vi "_add_attribute_name_to_error_message.vi"(7 "Attribute":T1={"Identifier"="", "Descriptive Name"="", "Data Type"=enum."Integer 32", "Command"="", "Access"=enum."Read/Write", "Range Table"="", "Read Callback"="", "Write Callback"="", "Supported Models"="", "Instrument Options"="", "Index"=0, "OPC Wait"=FALSE, "No Status Check"=FALSE, "Cache Only"=FALSE}, 8 "error in":errorcluster caption="error in (no error)", 10 "Recompose even if original message\nalready contains an attribute name (F)":bool, 11 "VISA resource name":refnum<visa-resource-name>) -> (0 "error out":errorcluster, 2 "Recomposed":bool, 3 "VISA resource name out":refnum<visa-resource-name>)   [LabVIEW 2022 SP3, in "hmp4000_rsidr_core.lvlib"]
uses:
  hmp4000_rsidr_core.lvlib
  type_Attribute.ctl
  type_Attribute_Data_Type.ctl
  type_ReadWriteAccess.ctl
  Trim Whitespace One-Sided.vi
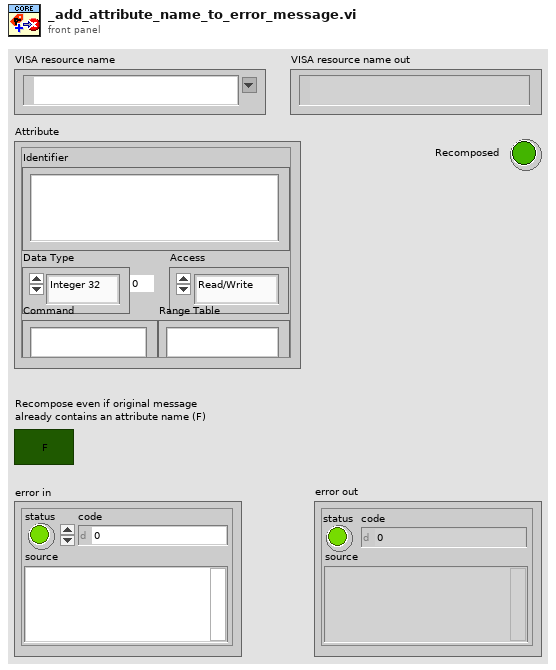
[diagram p1: front panel]
types:
  T1 = typedef "hmp4000_rsidr_core.lvlib/type_Attribute.ctl" = cluster{"Identifier":string, "Descriptive Name":string, "Data Type":T2, "Command":string, "Access":T3, "Range Table":string, "Read Callback":string, "Write Callback":string, "Supported Models":string, "Instrument Options":string, "Index":i32, "OPC Wait":bool, "No Status Check":bool, "Cache Only":bool}
  T2 = typedef "hmp4000_rsidr_core.lvlib/type_Attribute_Data_Type.ctl" = enum16{"Integer 32", "Double", "String", "Boolean", "None", "Integer 64", "RawString"}
  T3 = typedef "hmp4000_rsidr_core.lvlib/type_ReadWriteAccess.ctl" = enum16{"Read Only", "Write Only", "Read/Write"}
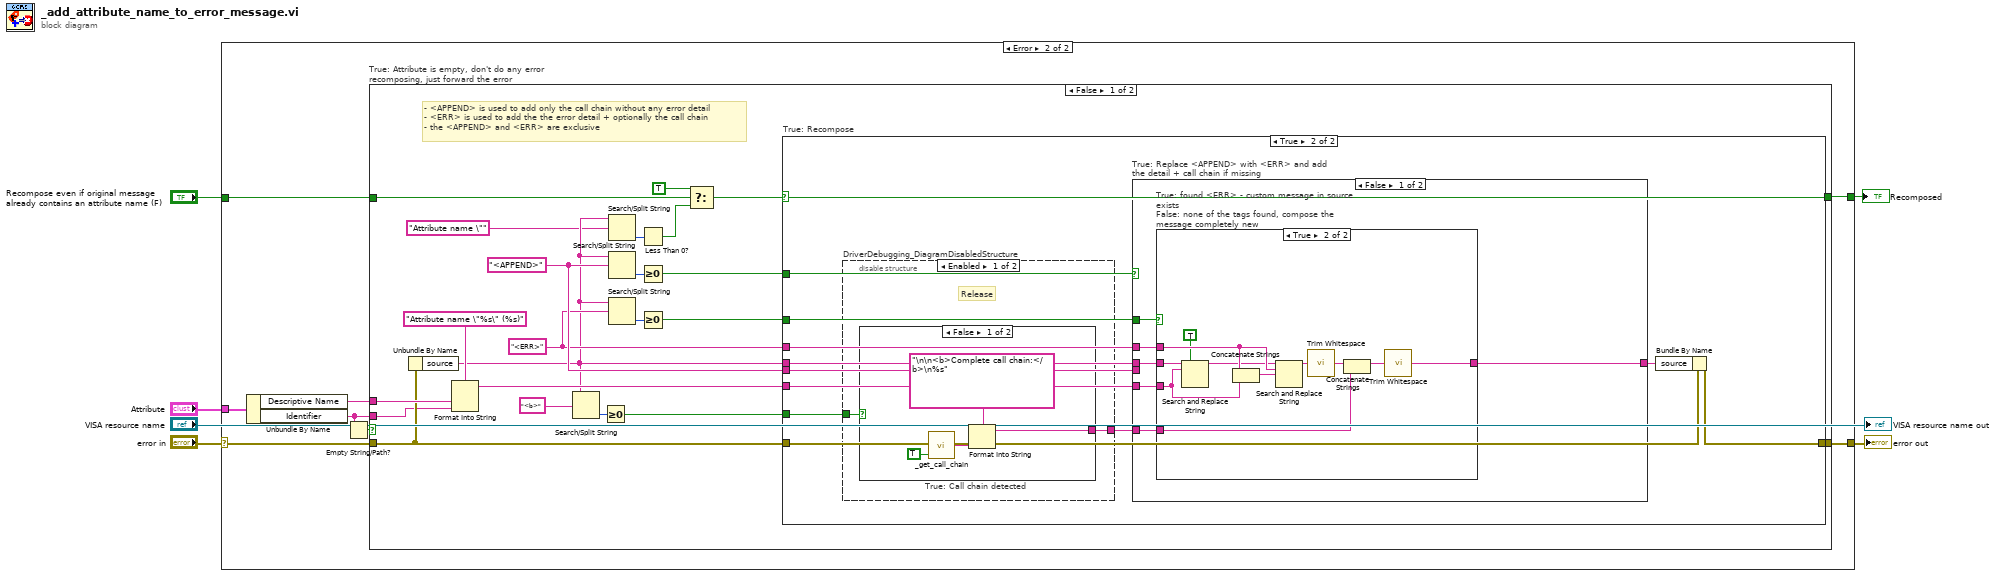
[diagram p0: block diagram]
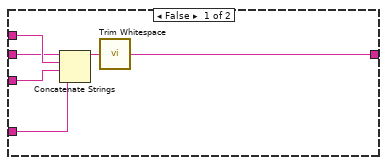
[diagram p6: hidden frame]
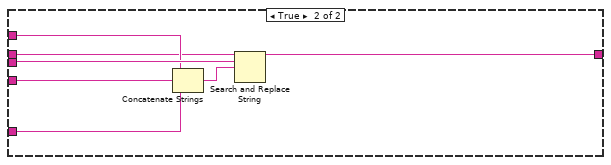
[diagram p7: hidden frame]
diagram:
  n1 = case shown="Error" "error in" {
    selector: "error in" -> [w7 w13]
    tunnel: [w7 w15] -> w6
    tunnel: "Attribute" -> [_ w10]
    tunnel: "Recompose even if original message\nalready contains an attribute name (F)" -> [_ w9]
    tunnel: [_ w8] -> w2
    frame No Error {
    }
    frame Error {
      n2 = Unbundle By Name(w10) -> ("Descriptive Name"=w14:string, "Identifier"=w11:string)
      n3 = Empty String/Path?(string/path=w11) -> (empty?=w12:bool)
      n4 = case "True: Attribute is empty, don't do any error recomposing, just forward the error" shown="False" w12 {
        tunnel: [w25 w86] -> w15
        tunnel: w11 -> [w16 _]
        tunnel: w14 -> [w32 _]
        tunnel: w13 -> [w26 w86]
        tunnel: w9 -> [w20 _]
        tunnel: [w17 _] -> w8
        frame False {
          w30 = "<ERR>" ("search string/char (-)")
          w31 = "<APPEND>" ("search string/char (-)")
          # "- <APPEND> is used to add only the call chain without any error detail\n- <ERR> is used to add the the error detail + optionally the call chain\n- the <APPEND> and <ERR> are exclusive"
          n5 = Unbundle By Name(w26) -> ("source"=w23:string)
          n6 = Format Into String(format string="Attribute name \"%s\" (%s)", w32, w16) -> (resulting string=w29:string)  [unwired: 2 in, 1 out]
          n7 = Search/Split String(string=w23, search string/char (-)="<b>" ("call chain beginning string")) -> (offset of match=w28:i32)  [unwired: 1 in, 2 out]
          n8 = Greater Or Equal To 0?(x=w28) -> (x >= 0?=w24:bool)
          n9 = Search/Split String(string=w23, search string/char (-)="Attribute name \"") -> (offset of match=w21:i32)  [unwired: 1 in, 2 out]
          n10 = Search/Split String(string=w23, search string/char (-)=w31) -> (offset of match=w37:i32)  [unwired: 1 in, 2 out]
          n11 = Search/Split String(string=w23, search string/char (-)=w30) -> (offset of match=w35:i32)  [unwired: 1 in, 2 out]
          n12 = Less Than 0?(x=w21) -> (x < 0?=w18:bool)
          n13 = Greater Or Equal To 0?(x=w37) -> (x >= 0?=w36:bool)
          n14 = Greater Or Equal To 0?(x=w35) -> (x >= 0?=w34:bool)
          n15 = Select(t=TRUE ("f"), s=w20, f=w18) -> (s? t:f=w17:bool)
          n16 = case "True: Recompose" shown="True" w17 {
            tunnel: w36 -> [_ w49]
            tunnel: w34 -> [_ w48]
            tunnel: w31 -> [_ w47]
            tunnel: w30 -> [_ w46]
            tunnel: w29 -> [_ w45]
            tunnel: w26 -> [w38 w43]
            tunnel: [w38 w42] -> w25
            tunnel: w24 -> [_ w41]
            tunnel: w23 -> [_ w39]
            frame False {
            }
            frame True {
              n17 = disable-structure "DriverDebugging_DiagramDisabledStructure" shown="Enabled" {
                disable-tunnel: w41 -> [w51 _]
                disable-tunnel: [w50 _] -> w40
                frame Enabled {
                  # "Release"
                  n18 = case "True: Call chain detected" shown="False" w51 {
                    tunnel: [w52 _] -> w50
                    frame False {
                      n19 = call "_get_call_chain.vi"("Remove lvlib names (F)"=TRUE) -> ("Call chain out in spreadsheet string"=w54:string)  [unwired: 2 in, 2 out]
                      n20 = Format Into String(format string="\n\n<b>Complete call chain:</b>\n%s", w54) -> (resulting string=w52:string)  [unwired: 2 in, 1 out]
                    }
                    frame True {
                    }
                  }
                }
                frame Disabled {
                  # "Debug"
                }
              }
              n21 = case "True: Replace <APPEND> with <ERR> and add the detail + call chain if missing" shown="False" w49 {
                tunnel: w48 -> [w61 _]
                tunnel: w39 -> [w60 w81]
                tunnel: w47 -> [_ w85]
                tunnel: w46 -> [w59 w84]
                tunnel: w45 -> [w58 w83]
                tunnel: [w57 w82] -> w44
                tunnel: w40 -> [w56 w79]
                frame False {
                  n22 = case "True: found <ERR> - custom message in source exists\nFalse: none of the tags found, compose the message completely new" shown="True" w61 {
                    tunnel: w60 -> [w64 w76]
                    tunnel: w59 -> [w66 w78]
                    tunnel: w58 -> [w65 w74]
                    tunnel: [w67 w77] -> w57
                    tunnel: w56 -> [w62 w72]
                    frame False {
                      n23 = Concatenate Strings(w64, w66, w65, w62) -> (w63:string)
                      n24 = call "Trim Whitespace.vi"("string"=w63) -> ("trimmed string"=w67:string)  [unwired: 1 in]
                    }
                    frame True {
                      n25 = Search and Replace String(replace all?=TRUE ("replace all? (F)"), input string=w76, search string=w74) -> (result string=w73:string)  [unwired: 5 in, 3 out]
                      n26 = Concatenate Strings(w78, w74) -> (w70:string)
                      n27 = Search and Replace String(input string=w73, search string=w78, replace string=w70) -> (result string=w71:string)  [unwired: 5 in, 3 out]
                      n28 = call "Trim Whitespace.vi"("string"=w71) -> ("trimmed string"=w69:string)  [unwired: 1 in]
                      n29 = Concatenate Strings(w69, w72) -> (w68:string)
                      n30 = call "Trim Whitespace.vi"("string"=w68) -> ("trimmed string"=w77:string)  [unwired: 1 in]
                    }
                  }
                }
                frame True {
                  n31 = Concatenate Strings(w84, w83, w79) -> (w80:string)
                  n32 = Search and Replace String(input string=w81, search string=w85, replace string=w80) -> (result string=w82:string)  [unwired: 5 in, 3 out]
                }
              }
              n33 = Bundle By Name(cluster=w43, "source"=w44) -> (w42:errorcluster)
            }
          }
        }
        frame True {
        }
      }
    }
  }
  "error out" <- w6
  "Recomposed" <- w2
  "VISA resource name out" <- "VISA resource name"
